vi "Create Client.vi"(8 "error in":errorcluster, 10 "Server Certificate File (.crt)":path, 11 "address":string) -> (0 "error out":errorcluster, 3 "gRPC ID Out":T1)   [LabVIEW 2021, in "CIFWaveformMonitorWrapper.lvlib"]
uses:
  CIFWaveformMonitorWrapper.lvlib
  <vilib>/gRPC/LabVIEW gRPC Library/grpc-lvsupport-release.lvlib
  CIFUtilities/CIFConfigurationFile/CIF Configuration File.lvlib
  CIFWaveformMonitor_server/CIFWaveformMonitor_server.lvlib
  <vilib>/gRPC/LabVIEW gRPC Library/Shared/grpcId.ctl
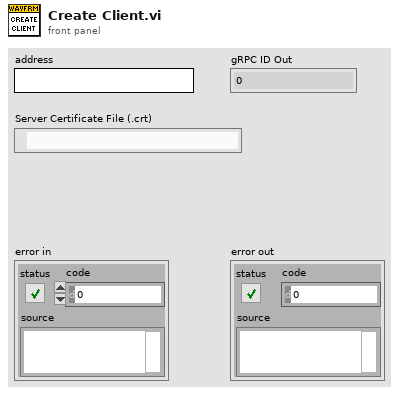
[diagram p1: front panel]
types:
  T1 = typedef "grpc-lvsupport-release.lvlib/grpcId.ctl" = u64
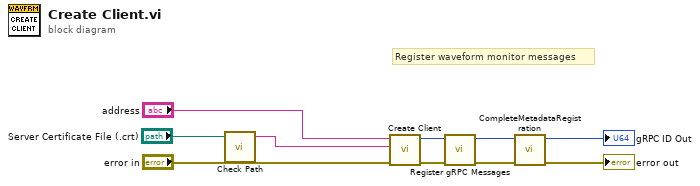
[diagram p0: block diagram]
diagram:
  # "Register waveform monitor messages"
  n1 = call "Check Path.vi"("path"="Server Certificate File (.crt)") -> ("Path String"=w3:string)  [unwired: 3 in]
  n2 = call <vilib>:"Create Client.vi"("error in"="error in", "certificatePath"=w3, "address"="address") -> ("error out"=w5:errorcluster, "ClientID out"=w6:T1)  [unwired: 7 in]
  n3 = call "Register gRPC Messages.vi"("error in (no error)"=w5, "gRPC ID"=w6) -> ("error out"=w2:errorcluster, "gRPC ID Out"=w1:T1)  [unwired: 8 in]
  n4 = call <vilib>:"CompleteMetadataRegistration.vi"("error in"=w2, "gRPC ID in"=w1) -> ("error out"=→"error out":errorcluster, "gRPC ID Out"=→"gRPC ID Out":T1)  [unwired: 8 in]
